vi "enqueue_data.vi"(0 "Active Analog Channel-Data Packages In":T1[](array[typedef]) {"Analog Input Channel"."Unit Conversion" format="%0.5f"; "Analog Input Channel"."TC Type" items=["J"=10072, "K"=10073, "N"=10077, "R"=10082, "S"=10085, "T"=10086, "B"=10047, "E"=10055]; "Analog Input Channel"."Sensor Offset" format="%0.5f"; "Analog Input Channel"."Sensor Max" format="%0.5f"; "Analog Input Channel"."Sensor Min" format="%0.5f"; "Analog Input Channel"."Maximum Value" format="%0.5f"; "Analog Input Channel"."Minimum Value" format="%0.5f"; "Analog Input Channel"."Terminal Configuration" items=["Default"=-1, "RSE"=10083, "NRSE"=10078, "Differential"=10106, "Pseudodifferential"=12529]}, 5 "Label indicies In":i32[](array[numeric]), 7 "Labels In":string[](array[string]), 9 "# of Samples":u32, 11 "error in":errorcluster, 12 "data Queue":refnum<queue>, 13 "Record dP Data":refnum<vi>, 14 "dP Recording Progress":refnum<vi>) -> (6 "Label indicies Out":i32[](array[numeric]), 8 "Labels Out":string[][](array[string]), 15 "error out":errorcluster)   [LabVIEW 2017]
uses:
  Box/Annular Flow/Jason/LabVIEW 2017/Input Channel Lists/analog_data_channel_pkg.ctl
  Input Channel Lists/input_channel.ctl
  Box/Annular Flow/Jason/LabVIEW 2017/Input Channel Lists/analog_data.ctl
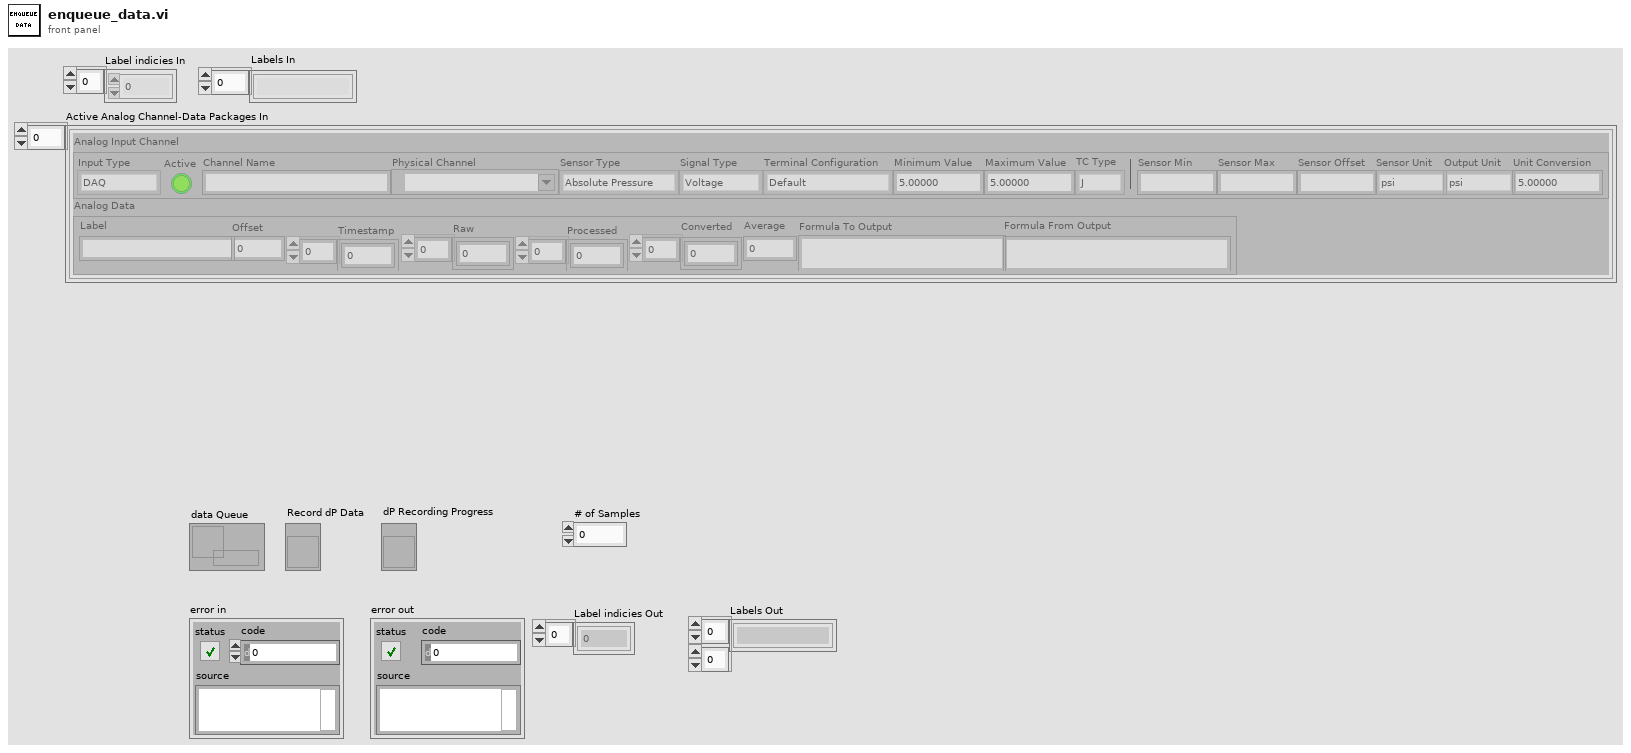
[diagram p1: front panel]
types:
  T1 = typedef "analog_data_channel_pkg.ctl" = cluster{"Analog Input Channel":T2, "Analog Data":T3}
  T2 = typedef "input_channel.ctl" = cluster{"Channel Name":string, "Physical Channel":tag, "Sensor Type":enum16{"Absolute Pressure", "Gauge Pressure", "Differential Pressure", "Temperature", "Mass Flow Rate", "Density", "Other"}, "Signal Type":enum16{"Voltage", "Current", "Temperature"}, "Terminal Configuration":i32, "Minimum Value":dbl, "Maximum Value":dbl, "TC Type":i32, "Sensor Min":dbl, "Sensor Max":dbl, "Sensor Offset":dbl, "Sensor Unit":enum16{"psi", "Pa", "inH2O", "inHg", "C", "K", "g/s", "g/cm3", "Volt", "Amp", ""}, "Output Unit":enum16{"psi", "Pa", "inH2O", "inHg", "C", "K", "g/s", "g/cm3", "Volt", "Amp", ""}, "Unit Conversion":dbl, "Active":bool, "Input Type":enum16{"DAQ", "Add-On"}}
  T3 = typedef "analog_data.ctl" = cluster{"Label":string, "Offset":dbl, "Timestamp":dbl[], "Raw":dbl[], "Processed":dbl[], "Converted":dbl[], "Average":dbl, "Formula To Output":string, "Formula From Output":string}
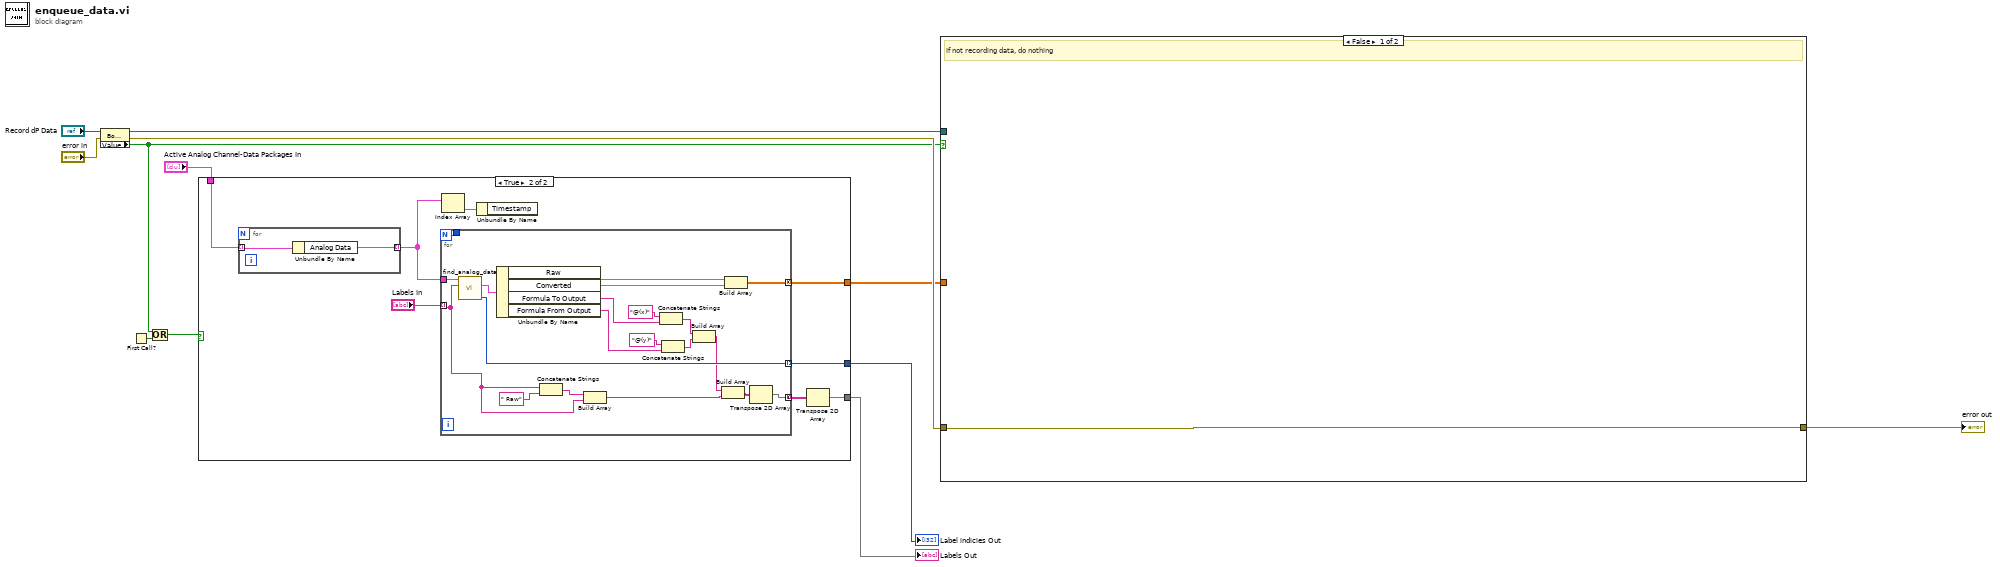
[diagram p0: block diagram]
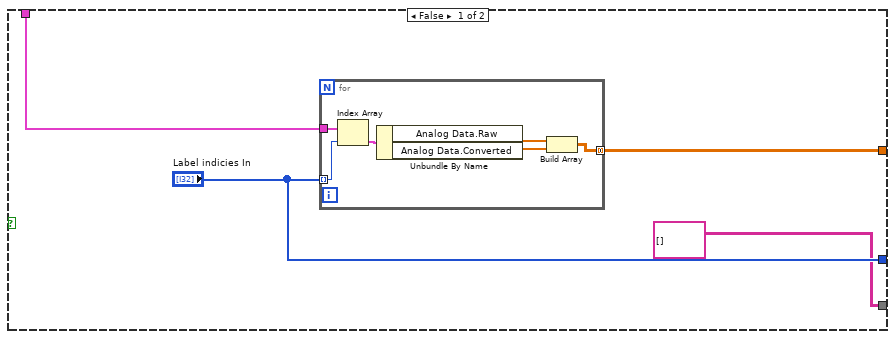
[diagram p2: hidden frame]
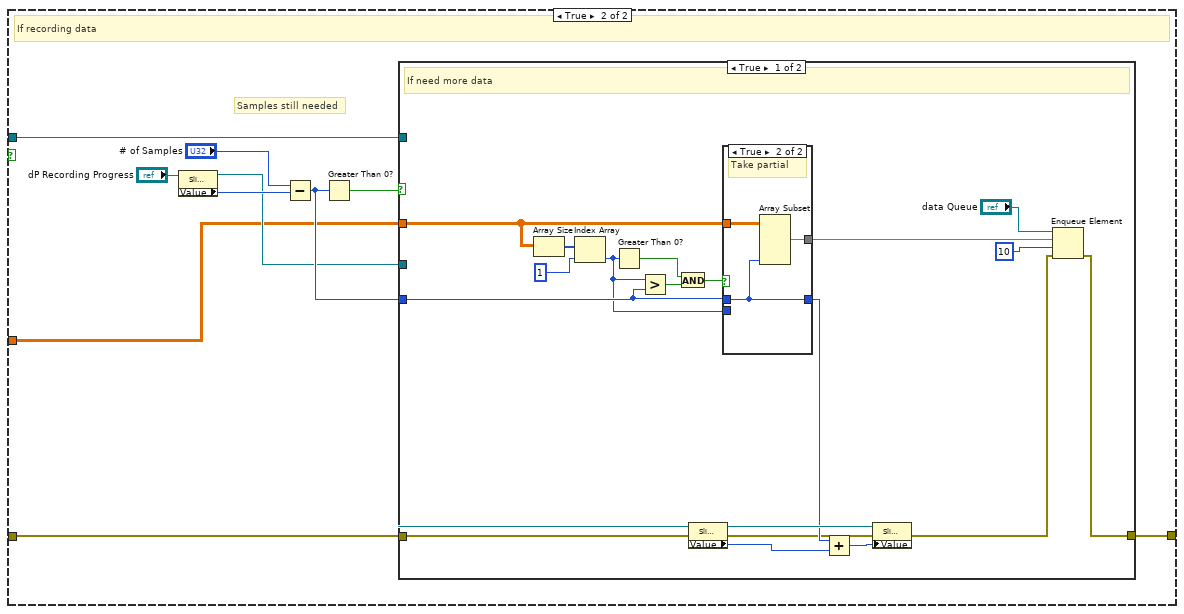
[diagram p3: hidden frame]
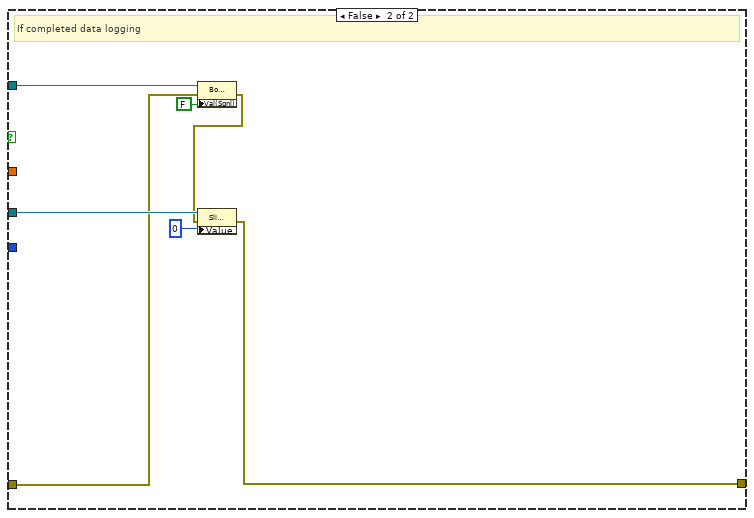
[diagram p5: hidden frame]
diagram:
  n1 = property class="Bool (strict)"(reference="Record dP Data", error in="error in") -> (reference out=w11:refnum<vi>, error out=w9:errorcluster, "Value"=w2:bool)
  n2 = First Call?() -> (First Call?: T/F=w3:bool)
  n3 = Or(x=w2, y=w3) -> (x .or. y?=w1:bool)
  n4 = case shown="True" w1 {
    tunnel: "Active Analog Channel-Data Packages In" -> [w15 w30]
    tunnel: [w16 w28] -> w7
    tunnel: ["Label indicies In" w27] -> w5
    tunnel: [string[][] [] w25] -> w6
    frame False {
      n5 = for {
        tunnel: [w22] -> w16 mode=concatenating
        tunnel: w15 -> [w19]
        tunnel: "Label indicies In" -> [w18] mode=indexing
        n6 = Index Array(array=w19, index=w18) -> (element=w17:T1)
        n7 = Unbundle By Name(w17) -> ("Analog Data.Raw"=w21:dbl[], "Analog Data.Converted"=w20:dbl[])
        n8 = Build Array(w21, w20) -> (w22:dbl[][])
      }
    }
    frame True {
      n9 = for {
        tunnel: w30 -> [w32] mode=indexing
        tunnel: [w31] -> w24 mode=indexing
        n10 = Unbundle By Name(w32) -> ("Analog Data"=w31:T3)
      }
      n11 = for {
        N -> [w33]
        tunnel: "Labels In" -> [w44] mode=indexing
        tunnel: w24 -> [w52]
        tunnel: [w51] -> w28 mode=concatenating
        tunnel: [w47] -> w27 mode=indexing
        tunnel: [w40] -> w26 mode=concatenating
        tunnel: [w33] -> _
        n12 = call "find_analog_data.vi"("Needle"=w44, "Haystack"=w52) -> ("Index"=w47:i32, "Needle Out"=w50:T3)  [unwired: 7 in, 1 out]
        n13 = Unbundle By Name(w50) -> ("Raw"=w49:dbl[], "Converted"=w48:dbl[], "Formula To Output"=w35:string, "Formula From Output"=w37:string)
        n14 = Concatenate Strings(w44, " Raw" ("string")) -> (w45:string)
        n15 = Build Array(w45, w44) -> (w43:string[])
        n16 = Concatenate Strings("@(x)" ("string"), w35) -> (w34:string)
        n17 = Concatenate Strings("@(y)" ("string"), w37) -> (w36:string)
        n18 = Build Array(w34, w36) -> (w42:string[])
        n19 = Build Array(w42, w43) -> (w41:string[][])
        n20 = Build Array(w49, w48) -> (w51:dbl[][])
        n21 = Transpose 2D Array(2D array=w41) -> (transposed array=w40:string[][])
      }
      n22 = Index Array(array=w24) -> (element=w23:T3)  [unwired: 1 in]
      n23 = Unbundle By Name(w23) -> ()  [unwired: 1 out]
      n24 = Transpose 2D Array(2D array=w26) -> (transposed array=w25:string[][])
    }
  }
  "Label indicies Out" <- w5
  "Labels Out" <- w6
  n25 = case shown="False" w2 {
    tunnel: w11 -> [_ w57]
    tunnel: [w53 w56] -> w10
    tunnel: w9 -> [w53 w55]
    tunnel: w7 -> [_ w54]
    frame False {
      # "If not recording data, do nothing"
    }
    frame True {
      # "Samples still needed"
      # "If recording data"
      n26 = property class="Slide (strict)"(reference="dP Recording Progress") -> (reference out=w58:refnum<vi>, "Value"=w62:u32)  [unwired: 1 in, 1 out]
      n27 = Subtract(x="# of Samples", y=w62) -> (x-y=w59:u32)
      n28 = Greater Than 0?(x=w59) -> (x > 0?=w60:bool)
      n29 = case shown="True" w60 {
        tunnel: w59 -> [w81 _]
        tunnel: w58 -> [w74 w93]
        tunnel: w57 -> [_ w92]
        tunnel: w54 -> [w69 _]
        tunnel: [w64 w90] -> w56
        tunnel: w55 -> [w66 w89]
        frame True {
          # "If need more data"
          n30 = Array Size(array=w69) -> (size(s)=w83:i32[])
          n31 = Index Array(array=w83, index=1) -> (element=w77:i32)
          n32 = Greater Than 0?(x=w77) -> (x > 0?=w80:bool)
          n33 = Greater?(x=w77, y=w81) -> (0:w79:bool)
          n34 = And(x=w80, y=w79) -> (x .and. y?=w78:bool)
          n35 = property class="Slide (strict)"(reference=w74, error in=w66) -> (reference out=w72:refnum<vi>, error out=w67:errorcluster, "Value"=w73:u32)
          n36 = case shown="True" w78 {
            tunnel: w69 -> [w85 w88]
            tunnel: w81 -> [_ w86]
            tunnel: [w85 w87] -> w68
            tunnel: [w84 w86] -> w70
            tunnel: w77 -> [w84 _]
            frame False {
              # "Take all"
            }
            frame True {
              # "Take partial"
              n37 = Array Subset(array=w88, length (col)=w86) -> (w87:dbl[][])  [unwired: 3 in]
            }
          }
          n38 = Add(x=w70, y=w73) -> (x+y=w71:u32)
          n39 = property class="Slide (strict)"(reference=w72, error in=w67, "Value"=w71) -> (error out=w65:errorcluster)  [unwired: 1 out]
          n40 = Enqueue Element(queue="data Queue", element=w68, timeout in ms (-1)=10, error in (no error)=w65) -> (error out=w64:errorcluster)  [unwired: 2 out]
        }
        frame False {
          # "If completed data logging"
          n41 = property class="Bool (strict)"(reference=w92, error in=w89, "Val(Sgnl)"=FALSE ("Value (Signaling)")) -> (error out=w91:errorcluster)  [unwired: 1 out]
          n42 = property class="Slide (strict)"(reference=w93, error in=w91, "Value"=u32 0 ("dP Recording Progress")) -> (error out=w90:errorcluster)  [unwired: 1 out]
        }
      }
    }
  }
  "error out" <- w10
